vi "Set - Signal Attribute.vi"(0 "reference in":refnum<class "GSwFormDSP.lvclass">, 5 "error in (no error)":errorcluster, 6 "wForm Attributes":T1="NI_ChannelName", 7 "Attribute":string[](array[string])) -> (14 "reference in":refnum<class "GSwFormDSP.lvclass">, 19 "error out":errorcluster)   [LabVIEW 2022 SP3, in "GSwFormDSP.lvclass"]
uses:
  GSwFormDSP.lvclass
  functions/Attribute List.ctl
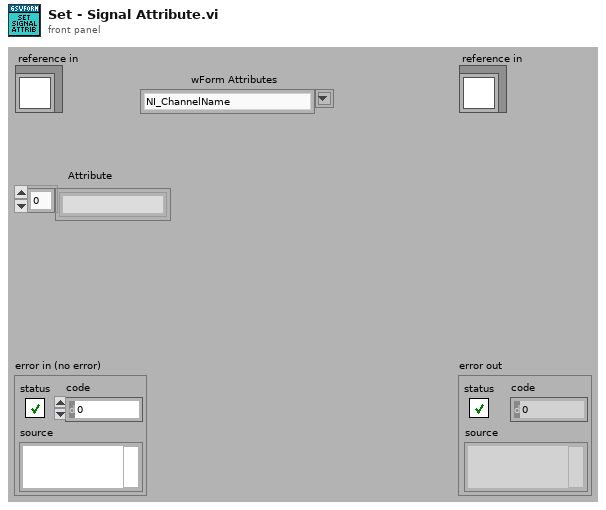
[diagram p1: front panel]
types:
  T1 = typedef "GSwFormDSP.lvclass/Attribute List.ctl" = string
  T2 = typedef "GSwFormDSP.lvclass/ObjectAttributesRef.ctl" = refnum<data-value>
  T3 = typedef "GSwFormDSP.lvclass/ObjectAttributes.ctl" = cluster{"Wform Ref":refnum<data-value>, "Nb Signals":i32, "Spectral Function Parameters":T4, "FFT":waveform(cdb)[], "Nb FFT":i32, "Nb Averages":i32[], "Reference Indexes":i32[], "Response Indexes":i32[], "Coherence":waveform(dbl)[], "TDF Parameters":T6, "DAQ":cluster{"Duration (sec)":dbl, "Buffer Size (Samples)":i32, "Offset (Samples)":i32}, "Filter Impulse Response (TDF)":waveform(dbl), "Sound Playback":T7}
  T4 = typedef "GSwFormDSP.lvclass/Spectral Parameters.ctl" = cluster{"Frequency resolution (Hz)":dbl, "Overlap":dbl, "Window":T5}
  T5 = typedef "NI_AALPro.lvlib/windowTd.ctl" = u32
  T6 = typedef "GSwFormDSP.lvclass/TDF Parameters.ctl" = cluster{"Filter":enum32{"Lowpass", "Highpass", "Bandpass", "Bandstop"}, "Type:":enum16{"Butterworth", "Chebyshev", "Inv Chebyshev", "Elliptic", "Bessel"}, "LP cutoff freq":dbl, "HP cutoff freq":dbl, "Order":i32, "passband ripple (dB)":dbl, "stopband attenuation (dB)":dbl, "Phaseless Filter":bool, "Include Fade IN and OUT":bool}
  T7 = typedef "GSwFormDSP.lvclass/Sound Playback.ctl" = cluster{"Timer start (ms)":u32, "task ID":T8, "Cursor Init Location (s)":dbl, "SC Volume":dbl}
  T8 = typedef "Sound Output Task ID.ctl" = u32
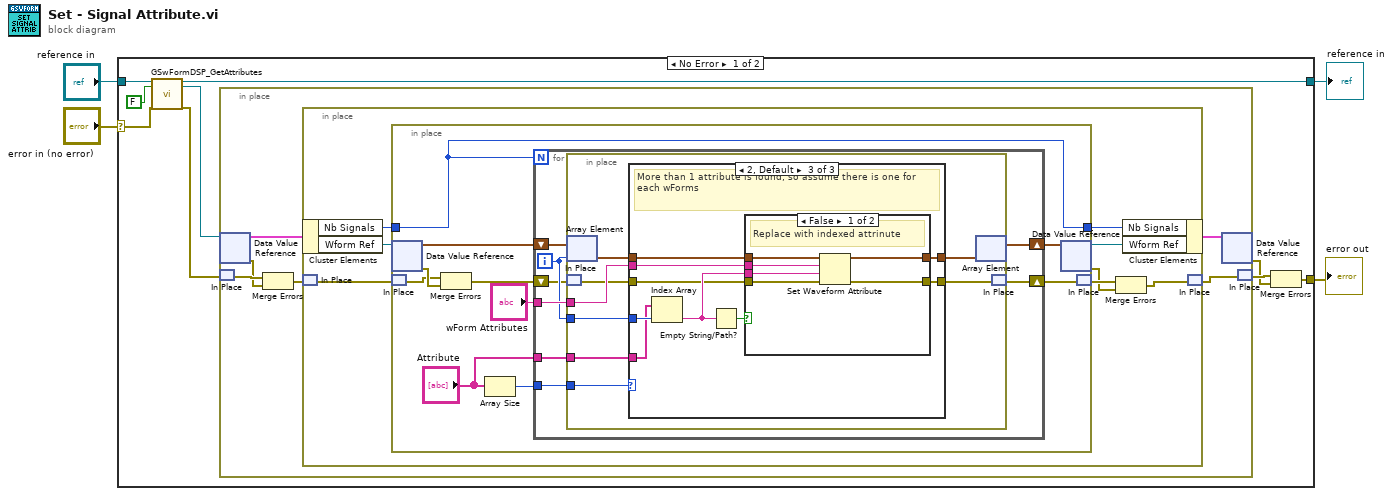
[diagram p0: block diagram]
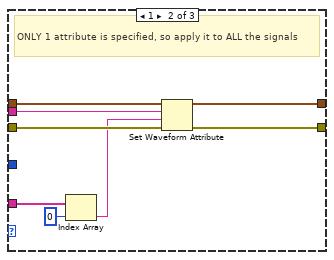
[diagram p3: hidden frame]
diagram:
  n1 = case shown="No Error" "error in (no error)" {
    selector: "error in (no error)" -> [w10 w82]
    tunnel: [w13 w82] -> w3
    tunnel: [w5 w81] -> w1
    tunnel: "reference in" -> [w11 w81]
    frame No Error {
      n2 = call "GSwFormDSP_GetAttributes.vi"("reference in"=w11, "return data? (T)"=FALSE, "error in (no error)"=w10) -> ("reference out"=w5:refnum<class "GSwFormDSP.lvclass">, "attributes ref"=w9:T2, "error out"=w8:errorcluster)  [unwired: 13 in, 1 out]
      n3 = in-place {
        n4 = in-place-dvr #1(w9) -> (w17:T3, w18:errorcluster)
        n5 = in-place-match #2(w8) -> (w19:errorcluster)
        n6 = Merge Errors(w19, w18) -> (w15:errorcluster)
        n7 = in-place {
          n8 = in-place-cluster #3(w17) -> ("Nb Signals"=w26:i32, "Wform Ref"=w27:refnum<data-value>)
          n9 = in-place-match #4(w15) -> (w25:errorcluster)
          n10 = in-place {
            in-place-border: w26 -> [w33]
            in-place-border: [w33] -> w23
            n11 = in-place-dvr #5(w27) -> (w37:waveform(dbl)[], w35:errorcluster)
            n12 = in-place-match #6(w25) -> (w34:errorcluster)
            n13 = Merge Errors(w34, w35) -> (w32:errorcluster)
            n14 = Array Size(array="Attribute") -> (size(s)=w29:i32)
            n15 = for {
              N: w33 -> [_]
              shift-right: [w44] -> w36
              shift-left: w37 -> [w45]
              tunnel: "wForm Attributes" -> [w43]
              shift-right: [w40] -> w31
              shift-left: w32 -> [w41]
              tunnel: w29 -> [w39]
              tunnel: "Attribute" -> [w38]
              i -> [w42]
              n16 = in-place {
                in-place-border: w43 -> [w52]
                in-place-border: w42 -> [w50]
                in-place-border: w39 -> [w47]
                in-place-border: w38 -> [w46]
                n17 = in-place-array #7(w45, w42) -> (w53:waveform(dbl))
                n18 = in-place-match #8(w41) -> (w49:errorcluster)
                n19 = case shown="2, Default" w47 {
                  tunnel: w53 -> [w55 w63 w71]
                  tunnel: w52 -> [_ w61 w70]
                  tunnel: [w55 w62 w69] -> w51
                  tunnel: w50 -> [_ _ w68]
                  tunnel: w49 -> [w54 w60 w66]
                  tunnel: [w54 w59 w65] -> w48
                  tunnel: w46 -> [_ w58 w64]
                  frame 0 {
                    # "NO attribute specified, so do nothing."
                  }
                  frame 1 {
                    # "ONLY 1 attribute is specified, so apply it to ALL the signals"
                    n20 = Index Array(array=w58, index=0) -> (element=w56:string)
                    n21 = Set Waveform Attribute(4:w60, 5:w56, 6:w61, 7:w63) -> (0:w59:errorcluster, 3:w62:waveform(dbl))  [unwired: 1 out]
                  }
                  frame 2, Default {
                    # "More than 1 attribute is found, so assume there is one for each wForms"
                    n22 = Index Array(array=w64, index=w68) -> (element=w67:string)
                    n23 = Empty String/Path?(string/path=w67) -> (empty?=w72:bool)
                    n24 = case shown="False" w72 {
                      tunnel: w67 -> [w75 _]
                      tunnel: w71 -> [w78 w80]
                      tunnel: w70 -> [w77 _]
                      tunnel: [w76 w80] -> w69
                      tunnel: w66 -> [w74 w79]
                      tunnel: [w73 w79] -> w65
                      frame False {
                        # "Replace with indexed attrinute"
                        n25 = Set Waveform Attribute(4:w74, 5:w75, 6:w77, 7:w78) -> (0:w73:errorcluster, 3:w76:waveform(dbl))  [unwired: 1 out]
                      }
                      frame True {
                        # "Empty, so do nothing"
                      }
                    }
                  }
                }
                n26 = in-place-array #7(w51) -> (w44:waveform(dbl)[])  [unwired: 1 out]
                n27 = in-place-match #8(w48) -> (w40:errorcluster)
              }
            }
            n28 = in-place-dvr #5(w36) -> (w24:refnum<data-value>, w21:errorcluster)
            n29 = in-place-match #6(w31) -> (w22:errorcluster)
          }
          n30 = Merge Errors(w22, w21) -> (w20:errorcluster)
          n31 = in-place-cluster #3("Nb Signals"=w23, "Wform Ref"=w24) -> (w16:T3)
          n32 = in-place-match #4(w20) -> (w14:errorcluster)
        }
        n33 = in-place-dvr #1(w16) -> (w6:errorcluster)  [unwired: 1 out]
        n34 = in-place-match #2(w14) -> (w7:errorcluster)
      }
      n35 = Merge Errors(w7, w6) -> (w13:errorcluster)
    }
    frame Error {
    }
  }
  "error out" <- w3
  "reference in" <- w1
